vi "Sparse2dArray.vi"() -> ()   [LabVIEW 2014]
uses:
  Private/Class/meth.Constructor.vi
  Private/Class/meth.Destructor.vi
  GLue.lvlib
panel:
  out "data":string[](array[string])
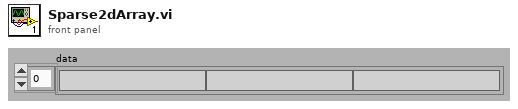
[diagram p1: front panel]
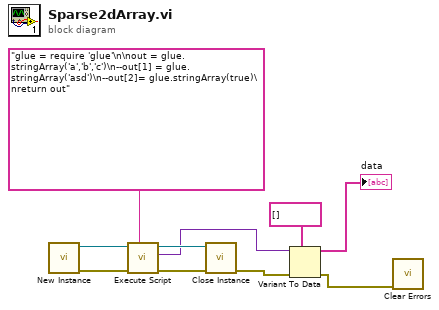
[diagram p0: block diagram]
diagram:
  n1 = call "New Instance.vi"() -> ("error out"=w6:errorcluster, "GLue out"=w7:refnum<class "class.GLue.lvclass">)  [unwired: 10 in]
  n2 = call "Execute Script.vi"("Script"="glue = require 'glue'\n\nout = glue.stringArray('a','b','c')\n--out[1] = glue.stringArray('asd')\n--out[2]= glue.stringArray(true)\nreturn out", "error in"=w6, "GLue in"=w7) -> ("error out"=w8:errorcluster, "Return Data"=w4:variant, "GLue out"=w9:refnum<class "class.GLue.lvclass">)  [unwired: 6 in]
  n3 = call "Close Instance.vi"("error in"=w8, "GLue in"=w9) -> ("error out"=w5:errorcluster)  [unwired: 9 in]
  n4 = Variant To Data(error in=w5, type=string[] [], Variant=w4) -> (data=→"data":string[], error out=w2:errorcluster)
  n5 = call <vilib>:"Clear Errors.vi"("error in (no error)"=w2) -> ()  [unwired: 5 in, 2 out]
